vi "Create File Directories.vi"(8 "error in (no error)":errorcluster) -> (0 "error out":errorcluster)   [LabVIEW 2018]
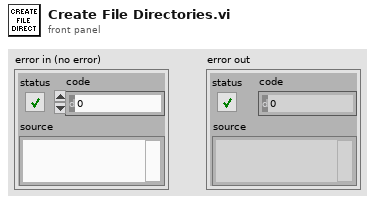
[diagram p1: front panel]
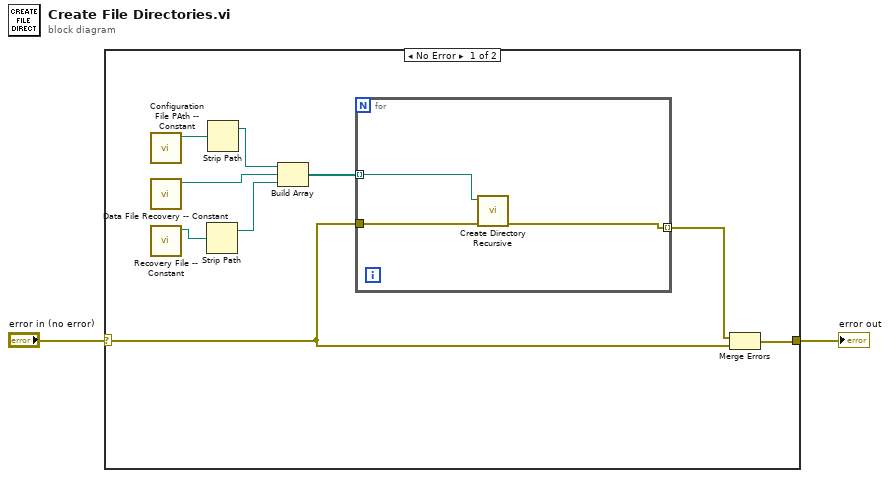
[diagram p0: block diagram]
diagram:
  n1 = case shown="No Error" "error in (no error)" {
    selector: "error in (no error)" -> [w7 w15]
    tunnel: [w9 w15] -> w1
    frame No Error {
      n2 = call "Configuration File PAth -- Constant.vi"() -> ("Configuration File Path"=w11:path)  [unwired: 11 in]
      n3 = call "Data File Recovery -- Constant.vi"() -> ("Data File Directory"=w5:path)  [unwired: 11 in]
      n4 = call "Recovery File -- Constant.vi"() -> ("Recovery File Path"=w4:path)  [unwired: 11 in]
      n5 = Strip Path(path=w4) -> (stripped path=w3:path)  [unwired: 1 out]
      n6 = Strip Path(path=w11) -> (stripped path=w10:path)  [unwired: 1 out]
      n7 = Build Array(w10, w5, w3) -> (w6:path[])
      n8 = for {
        tunnel: [w13] -> w8 mode=indexing
        tunnel: w7 -> [w14]
        tunnel: w6 -> [w12] mode=indexing
        n9 = call <vilib>:"Create Directory Recursive.vi"("error in (no error)"=w14, "directory"=w12) -> ("error out"=w13:errorcluster)  [unwired: 3 in, 2 out]
      }
      n10 = Merge Errors(w8, w7) -> (w9:errorcluster)
    }
    frame Error {
    }
  }
  "error out" <- w1
